vi "Byte Buffer.Get Size.vi"(8 "error in (no error)":errorcluster, 11 "Byte Buffer in":refnum<class "Byte Buffer.lvclass">) -> (0 "error out":errorcluster, 2 "size":i32, 3 "Byte Buffer out":refnum<class "Byte Buffer.lvclass">)   [LabVIEW 2016, in "VeriStand Data.lvlib" / "Byte Buffer.lvclass"]
doc: "Returns the current size of the provided <B>buffer</B>."
uses:
  Byte Buffer.lvclass
  Byte Buffer.lvclass/Byte Buffer.ctl
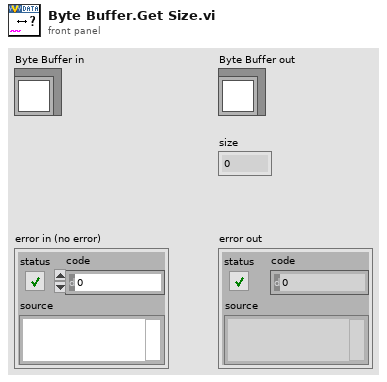
[diagram p1: front panel]
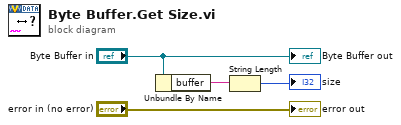
[diagram p0: block diagram]
diagram:
  n1 = Unbundle By Name("Byte Buffer in") -> ("buffer"=w2:string)
  n2 = String Length(string=w2) -> (length=→"size":i32)
  "error out" <- "error in (no error)"
  "Byte Buffer out" <- "Byte Buffer in"
